vi "DestroySingletonRef.vi"(8 "error in (no error)":errorcluster, 11 "DVR":refnum<data-value>) -> (0 "error out":errorcluster)   [LabVIEW 2017, in "TimerEngine.lvlib" / "TimerEngine.lvclass"]
uses:
  TimerEngine.lvclass
  TimerEngine.lvclass/TimerEngine.ctl
  _TimerClass/Timer.lvclass
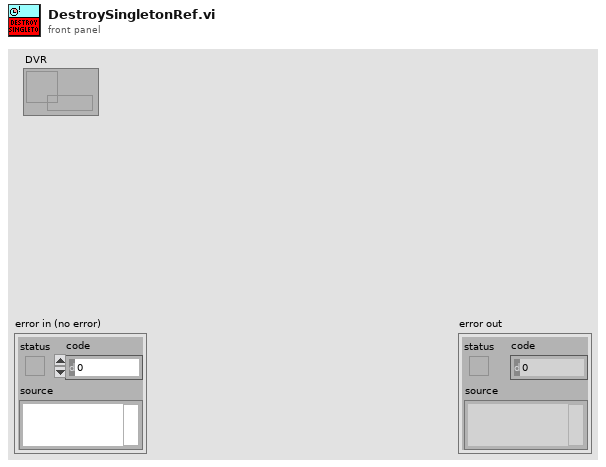
[diagram p1: front panel]
types:
  T1 = typedef "TimerEngine.lvlib/TimerEngine.lvclass/WatchDog--QueueRef.ctl" = refnum<queue>
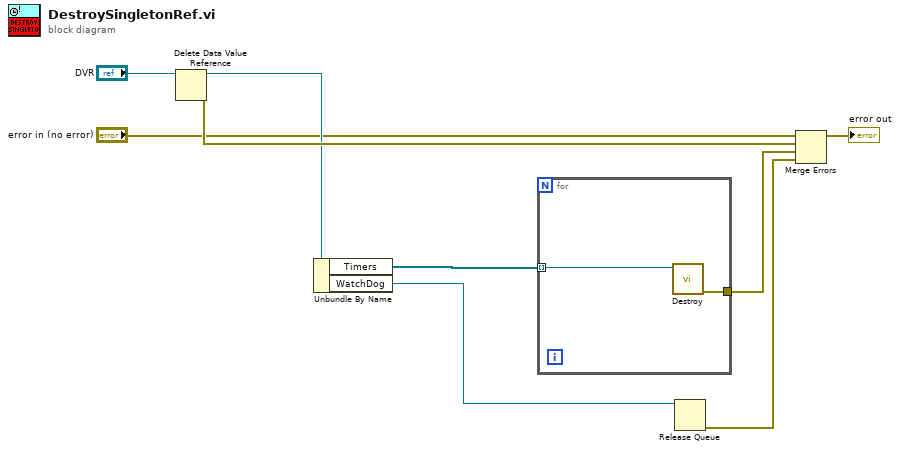
[diagram p0: block diagram]
diagram:
  n1 = Delete Data Value Reference(data value reference="DVR") -> (data value=w7:refnum<class "TimerEngine.lvclass">, error out=w8:errorcluster)  [unwired: 1 in]
  n2 = Unbundle By Name(w7) -> ("Timers"=w1:refnum<class "Timer.lvclass">[], "WatchDog"=w3:T1)
  n3 = for {
    tunnel: [w11] -> w5
    tunnel: w1 -> [w10] mode=indexing
    n4 = call "Destroy.vi"("Timer in"=w10) -> ("error out"=w11:errorcluster)  [unwired: 9 in, 1 out]
  }
  n5 = Release Queue(queue=w3) -> (error out=w2:errorcluster)  [unwired: 2 in, 2 out]
  n6 = Merge Errors("error in (no error)", w8, w5, w2) -> (→"error out":errorcluster)
